vi "Buffer Event Data.vi"(8 "error in":errorcluster, 10 "Path":path, 11 "TDMS in":refnum<class "TDMS.lvclass">) -> (0 "error out":errorcluster, 3 "TDMS out":refnum<class "TDMS.lvclass">)   [LabVIEW 2019, in "TDMS.lvlib" / "TDMS.lvclass"]
uses:
  TDMS.lvclass
  TDMS.lvclass/TDMS.ctl
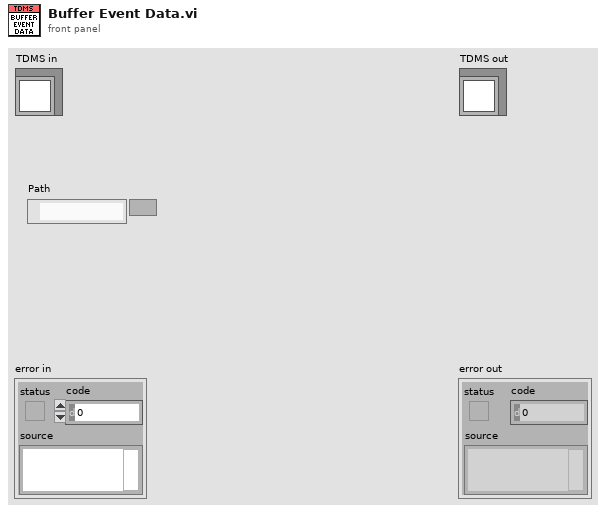
[diagram p1: front panel]
types:
  T1 = cluster{"Time":timestamp[], "Instrument":string[], "Description":string[], "Data":string[]}
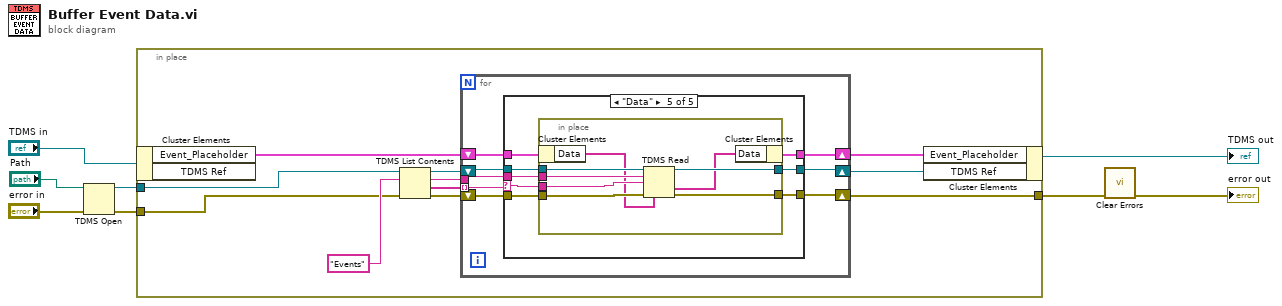
[diagram p0: block diagram]
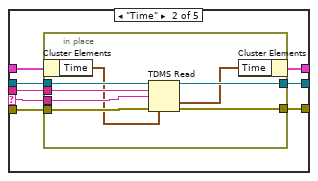
[diagram p3: hidden frame]
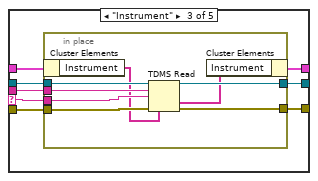
[diagram p4: hidden frame]
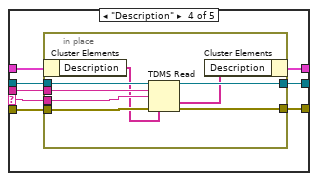
[diagram p5: hidden frame]
diagram:
  n1 = TDMS Open(8:"error in", 11:"Path") -> (0:w5:errorcluster, 3:w3:refnum<k34>)  [unwired: 5 in]
  n2 = in-place {
    in-place-border: w5 -> [w14]
    in-place-border: [w12] -> w6
    in-place-border: w3 -> [w9]
    n3 = in-place-cluster #1("TDMS in") -> ("Event_Placeholder"=w11:T1)  [unwired: 1 out]
    n4 = TDMS List Contents(4:w14, 6:"Events" ("group name"), 7:w9) -> (0:w17:errorcluster, 1:w16:string[], 2:w15:string, 3:w18:refnum<k34>)
    n5 = for {
      shift-right: [w24] -> w13
      shift-left: w18 -> [w27]
      tunnel: w16 -> [w20] mode=indexing
      tunnel: w15 -> [w23]
      shift-right: [w25] -> w12
      shift-left: w17 -> [w26]
      shift-right: [w21] -> w10
      shift-left: w11 -> [w22]
      n6 = case shown="\"Data\"" w20 {
        selector: w20 -> [_ w31 w47 w63 w79]
        tunnel: w27 -> [w29 w38 w54 w70 w86]
        tunnel: w26 -> [w28 w37 w53 w69 w85]
        tunnel: [w28 w36 w52 w68 w84] -> w25
        tunnel: [w29 w35 w51 w67 w83] -> w24
        tunnel: w23 -> [_ w34 w50 w66 w82]
        tunnel: w22 -> [w30 w33 w49 w65 w81]
        tunnel: [w30 w32 w48 w64 w80] -> w21
        frame "False", Default {
        }
        frame "Time" {
          n7 = in-place {
            in-place-border: w38 -> [w46]
            in-place-border: w37 -> [w45]
            in-place-border: [w44] -> w36
            in-place-border: [w43] -> w35
            in-place-border: w34 -> [w42]
            in-place-border: w31 -> [w41]
            n8 = in-place-cluster #2(w33) -> ("Time"=w40:timestamp[])
            n9 = TDMS Read(0:w46, 5:w42, 7:w41, 11:w45, 12:w40) -> (4:w43:refnum<k34>, 10:w39:timestamp[], 15:w44:errorcluster)  [unwired: 3 in, 3 out]
            n10 = in-place-cluster #2("Time"=w39) -> (w32:T1)
          }
        }
        frame "Instrument" {
          n11 = in-place {
            in-place-border: w54 -> [w62]
            in-place-border: w53 -> [w61]
            in-place-border: [w60] -> w52
            in-place-border: [w59] -> w51
            in-place-border: w50 -> [w58]
            in-place-border: w47 -> [w57]
            n12 = in-place-cluster #3(w49) -> ("Instrument"=w56:string[])
            n13 = TDMS Read(0:w62, 5:w58, 7:w57, 11:w61, 12:w56) -> (4:w59:refnum<k34>, 10:w55:string[], 15:w60:errorcluster)  [unwired: 3 in, 3 out]
            n14 = in-place-cluster #3("Instrument"=w55) -> (w48:T1)
          }
        }
        frame "Description" {
          n15 = in-place {
            in-place-border: w70 -> [w78]
            in-place-border: w69 -> [w77]
            in-place-border: [w76] -> w68
            in-place-border: [w75] -> w67
            in-place-border: w66 -> [w74]
            in-place-border: w63 -> [w73]
            n16 = in-place-cluster #4(w65) -> ("Description"=w72:string[])
            n17 = TDMS Read(0:w78, 5:w74, 7:w73, 11:w77, 12:w72) -> (4:w75:refnum<k34>, 10:w71:string[], 15:w76:errorcluster)  [unwired: 3 in, 3 out]
            n18 = in-place-cluster #4("Description"=w71) -> (w64:T1)
          }
        }
        frame "Data" {
          n19 = in-place {
            in-place-border: w86 -> [w94]
            in-place-border: w85 -> [w93]
            in-place-border: [w92] -> w84
            in-place-border: [w91] -> w83
            in-place-border: w82 -> [w90]
            in-place-border: w79 -> [w89]
            n20 = in-place-cluster #5(w81) -> ("Data"=w88:string[])
            n21 = TDMS Read(0:w94, 5:w90, 7:w89, 11:w93, 12:w88) -> (4:w91:refnum<k34>, 10:w87:string[], 15:w92:errorcluster)  [unwired: 3 in, 3 out]
            n22 = in-place-cluster #5("Data"=w87) -> (w80:T1)
          }
        }
      }
    }
    n23 = in-place-cluster #1("Event_Placeholder"=w10, "TDMS Ref"=w13) -> (→"TDMS out":refnum<class "TDMS.lvclass">)
  }
  n24 = call <vilib>:"Clear Errors.vi"("error in (no error)"=w6) -> ("error out"=→"error out":errorcluster)  [unwired: 5 in, 1 out]
